vi "Get Error Details (Error 1097).vi"(11 "error":errorcluster) -> (1 "Message":string, 2 "Stack Trace":string, 3 "Type":string)   [LabVIEW 2013, in "JUnit Conversion.lvlib"]
uses:
  JUnit Conversion.lvlib
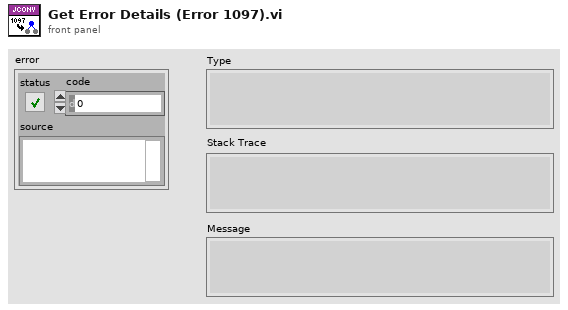
[diagram p1: front panel]
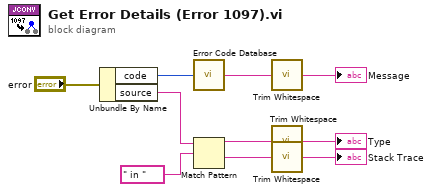
[diagram p0: block diagram]
diagram:
  n1 = Unbundle By Name("error") -> ("code"=w2:i32, "source"=w1:string)
  n2 = call <vilib>:"Error Code Database.vi"("Error Code"=w2) -> ("Error Text"=w7:string)
  n3 = Match Pattern(string=w1, regular expression=" in ") -> (before substring=w9:string, after substring=w8:string)  [unwired: 1 in, 2 out]
  n4 = call <vilib>:"Trim Whitespace.vi"("string"=w7) -> ("trimmed string"=→"Message":string)  [unwired: 1 in]
  n5 = call <vilib>:"Trim Whitespace.vi"("string"=w9) -> ("trimmed string"=→"Type":string)  [unwired: 1 in]
  n6 = call <vilib>:"Trim Whitespace.vi"("string"=w8) -> ("trimmed string"=→"Stack Trace":string)  [unwired: 1 in]
